vi "Example_MoveWithIPM.vi"() -> ()   [LabVIEW 2018]
doc: "Example how to do a interpolated position movement. Before starts this example the device must be tuned and the parameter settings must be correct.\nThe example shows:\n - how to initialise and close an interface (e.g. USB)\n - define home position to 0\n - sequence of an interpolated positioning (sinus wave untill stop button is pressed)\n - stops the trajectory"
panel:
  in  "stop":bool
  in  "array for PVT values":T1(array[cluster])=[{"position"=1492, "velocity"=203, "time"=240}, {"position"=2891, "velocity"=184, "time"=240}, {"position"=4107, "velocity"=153, "time"=240}, {"position"=5066, "velocity"=112, "time"=240}, {"position"=5706, "velocity"=65, "time"=240}, {"position"=5988, "velocity"=13, "time"=240}, {"position"=5894, "velocity"=-39, "time"=240}, {"position"=5429, "velocity"=-89, "time"=240}, {"position"=4623, "velocity"=-134, "time"=240}, {"position"=3527, "velocity"=-169, "time"=240}, {"position"=2209, "velocity"=-195, "time"=240}, {"position"=752, "velocity"=-208, "time"=240}, {"position"=-752, "velocity"=-208, "time"=240}, {"position"=-2209, "velocity"=-195, "time"=240}, {"position"=-3527, "velocity"=-169, "time"=240}, {"position"=-4623, "velocity"=-134, "time"=240}, {"position"=-5429, "velocity"=-89, "time"=240}, {"position"=-5894, "velocity"=-39, "time"=240}, {"position"=-5988, "velocity"=13, "time"=240}, {"position"=-5706, "velocity"=65, "time"=240}, {"position"=-5066, "velocity"=112, "time"=240}, {"position"=-4107, "velocity"=153, "time"=240}, {"position"=-2891, "velocity"=184, "time"=240}, {"position"=-1492, "velocity"=203, "time"=240}, {"position"=0, "velocity"=209, "time"=240}, {"position"=1492, "velocity"=203, "time"=240}, {"position"=2891, "velocity"=184, "time"=240}, {"position"=4107, "velocity"=153, "time"=240}, {"position"=5066, "velocity"=112, "time"=240}, {"position"=5706, "velocity"=65, "time"=240}, {"position"=5988, "velocity"=13, "time"=240}, {"position"=5894, "velocity"=-39, "time"=240}, {"position"=5429, "velocity"=-89, "time"=240}, {"position"=4623, "velocity"=-134, "time"=240}, {"position"=3527, "velocity"=-169, "time"=240}, {"position"=2209, "velocity"=-195, "time"=240}, {"position"=752, "velocity"=-208, "time"=240}, {"position"=-752, "velocity"=-208, "time"=240}, {"position"=-2209, "velocity"=-195, "time"=240}, {"position"=-3527, "velocity"=-169, "time"=240}, {"position"=-4623, "velocity"=-134, "time"=240}, {"position"=-5429, "velocity"=-89, "time"=240}, {"position"=-5894, "velocity"=-39, "time"=240}, {"position"=-5988, "velocity"=13, "time"=240}, {"position"=-5706, "velocity"=65, "time"=240}, {"position"=-5066, "velocity"=112, "time"=240}, {"position"=-4107, "velocity"=153, "time"=240}, {"position"=-2891, "velocity"=184, "time"=240}, {"position"=-1492, "velocity"=203, "time"=204}, {"position"=0, "velocity"=209, "time"=240}, {"position"=1492, "velocity"=203, "time"=240}, {"position"=2891, "velocity"=184, "time"=240}, {"position"=4107, "velocity"=153, "time"=240}, {"position"=5066, "velocity"=112, "time"=240}, {"position"=5706, "velocity"=65, "time"=240}, {"position"=5988, "velocity"=13, "time"=240}, {"position"=5894, "velocity"=-39, "time"=240}, {"position"=5429, "velocity"=-89, "time"=240}, {"position"=4623, "velocity"=-134, "time"=240}, {"position"=3527, "velocity"=-169, "time"=240}, {"position"=2209, "velocity"=-195, "time"=240}, {"position"=752, "velocity"=-208, "time"=240}, {"position"=-752, "velocity"=-208, "time"=240}, {"position"=-2209, "velocity"=-195, "time"=240}, {"position"=-3527, "velocity"=-169, "time"=240}, {"position"=-4623, "velocity"=-134, "time"=240}, {"position"=-5429, "velocity"=-89, "time"=240}, {"position"=-5894, "velocity"=-39, "time"=240}, {"position"=-5988, "velocity"=13, "time"=240}, {"position"=-5706, "velocity"=65, "time"=240}, {"position"=-5066, "velocity"=112, "time"=240}, {"position"=-4106, "velocity"=153, "time"=240}, {"position"=-2891, "velocity"=184, "time"=240}, {"position"=-1492, "velocity"=203, "time"=240}, {"position"=0, "velocity"=209, "time"=240}]
  in  "IPM buffer parameter":T2={"underflowWarningLimit"=4, "overflowWarningLimit"=60}
  in  "nodeId":u16=1
  in  "communication settings in":T3={"deviceName"="EPOS2", "protocolStackName"="MAXON SERIAL V2", "interfaceName"="USB", "portName"="USB0", "baudrate"=1000000, "timeout"=500}
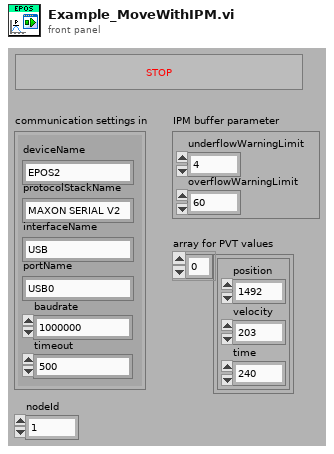
[diagram p1: front panel]
types:
  T1 = cluster{"position":i32, "velocity":i32, "time":u8}[]
  T2 = cluster{"underflowWarningLimit":u16, "overflowWarningLimit":u16}
  T3 = cluster{"deviceName":string, "protocolStackName":string, "interfaceName":string, "portName":string, "baudrate":u32, "timeout":u32}
  T4 = cluster{"position":i32, "velocity":i32, "time":u8}
  T5 = cluster{"trajectoryRunning":i32, "isUnderflowWarning":i32, "isOverflowWarning":i32, "isVelocityWarning":i32, "isAccelerationWarning":i32, "isUnderflowError":i32, "isOverflowError":i32, "isVelocityError":i32, "isAccelerationError":i32}
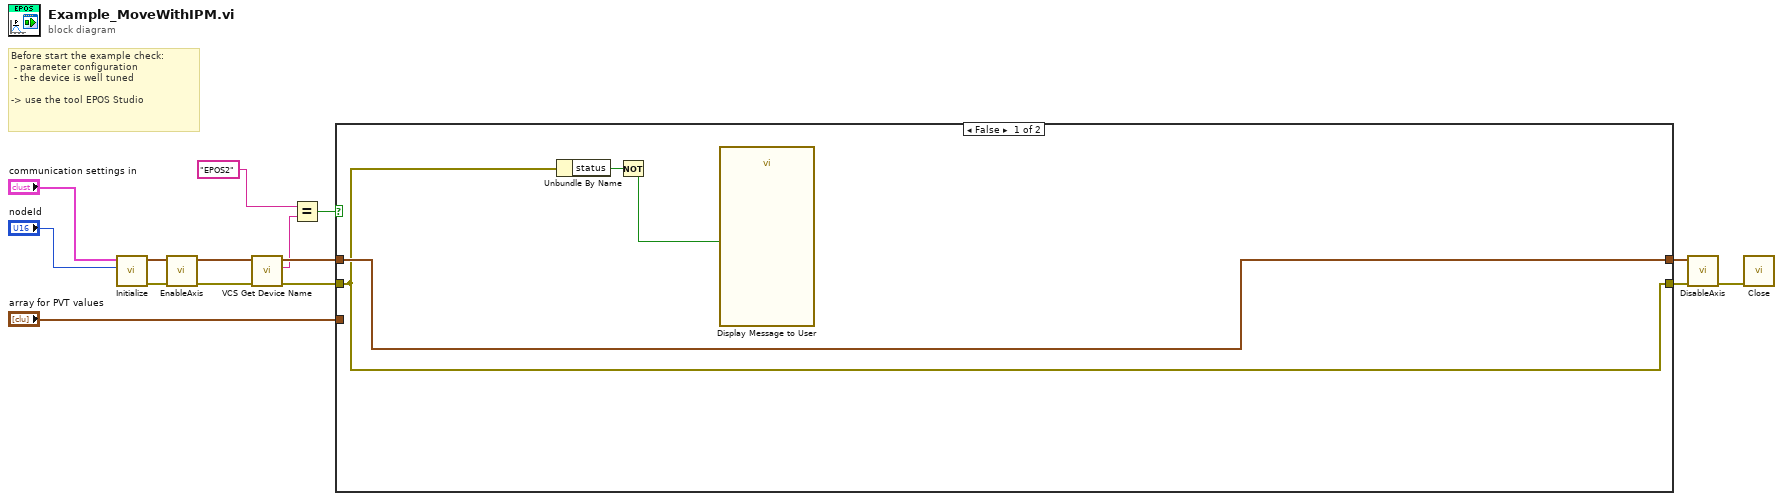
[diagram p0: block diagram]
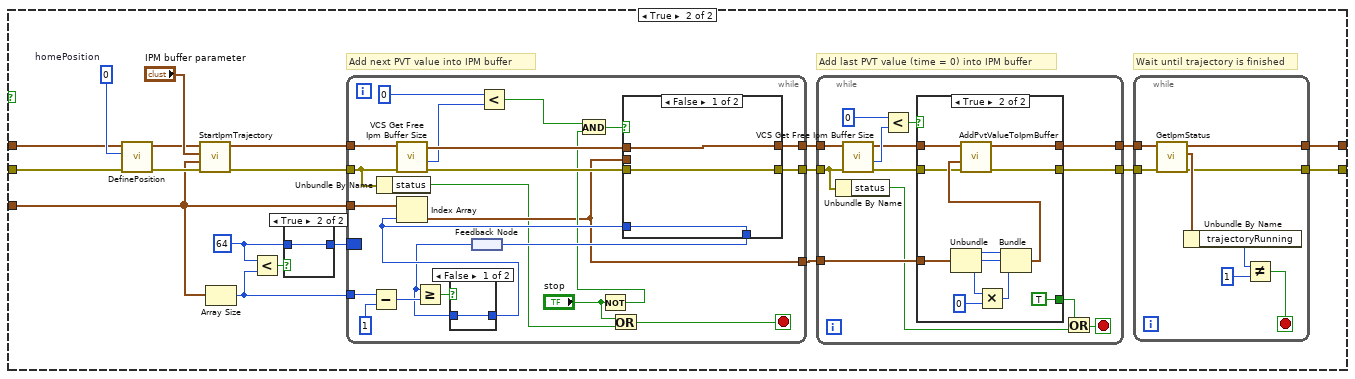
[diagram p2: hidden frame]
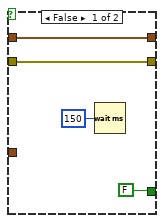
[diagram p3: hidden frame]
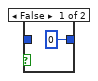
[diagram p4: hidden frame]
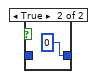
[diagram p5: hidden frame]
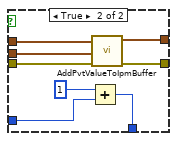
[diagram p6: hidden frame]
diagram:
  # "Before start the example check:\n - parameter configuration\n - the device is well tuned \n\n-> use the tool EPOS Studio"
  n1 = call "Initialize.vi"("nodeId"="nodeId", "communication settings in"="communication settings in") -> ("error out"=w13:errorcluster, "axis out"=w12:cluster{"keyHandle":u32, "nodeId":u16})  [unwired: 8 in]
  n2 = call "EnableAxis.vi"("error in (no error)"=w13, "axis in"=w12) -> ("error out"=w5:errorcluster, "axis out"=w4:cluster{"keyHandle":u32, "nodeId":u16})  [unwired: 4 in]
  n3 = call "VCS Get Device Name.vi"("error in (no error)"=w5, "axis in"=w4) -> ("error out"=w6:errorcluster, "deviceName"=w2:string, "axis out"=w7:cluster{"keyHandle":u32, "nodeId":u16})  [unwired: 7 in]
  n4 = Equal?(x="EPOS2", y=w2) -> (x = y?=w3:bool)
  n5 = case shown="False" w3 {
    tunnel: "array for PVT values" -> [_ w35]
    tunnel: [w17 w28] -> w9
    tunnel: [w16 w27] -> w8
    tunnel: w7 -> [w17 w21]
    tunnel: w6 -> [w16 w20]
    frame False {
      n6 = Unbundle By Name(w16) -> ("status"=w18:bool)
      n7 = Not(x=w18) -> (.not. x?=w19:bool)
      n8 = call "Display Message to User"("Enable"=w19) -> ()  [unwired: 9 in, 2 out]
    }
    frame True {
      w29 = 64 ("x")
      w39 = 0  # homePosition
      # "Wait until trajectory is finished"
      # "Add last PVT value (time = 0) into IPM buffer"
      # "Add next PVT value into IPM buffer"
      n9 = call "DefinePosition.vi"("error in (no error)"=w20, "homePosition"=w39, "axis in"=w21) -> ("error out"=w37:errorcluster, "axis out"=w36:cluster{"keyHandle":u32, "nodeId":u16})  [unwired: 3 in]
      n10 = call "StartIpmTrajectory.vi"("error in (no error)"=w37, "array for PVT values (max. 64 values)"=w35, "IPM buffer parameter"="IPM buffer parameter", "axis in"=w36) -> ("error out"=w33:errorcluster, "axis out"=w34:cluster{"keyHandle":u32, "nodeId":u16})  [unwired: 2 in]
      n11 = Array Size(array=w35) -> (size(s)=w32:i32)
      n12 = Less?(x=w29, y=w32) -> (x < y?=w31:bool)
      n13 = case shown="True" w31 {
        tunnel: [0 ("x") w78] -> w30
        tunnel: w29 -> [_ w78]
        frame False {
        }
        frame True {
        }
      }
      n14 = while {
        tunnel: w35 -> [w101]
        tunnel: w32 -> [w91]
        tunnel: [w99] -> w26
        tunnel: [w98] -> w25
        tunnel: w34 -> [w96]
        tunnel: w33 -> [w82]
        tunnel: [w83] -> w24
        border: w30 -> [_]
        stop <- w79 stop-if-true
        n15 = Subtract(x=w91, y=1) -> (x-y=w95:i32)
        n16 = Unbundle By Name(w82) -> ("status"=w80:bool)
        n17 = call "VCS Get Free Ipm Buffer Size.vi"("error in (no error)"=w82, "axis in"=w96) -> ("error out"=w97:errorcluster, "bufferSize"=w87:u32, "axis out"=w100:cluster{"keyHandle":u32, "nodeId":u16})  [unwired: 6 in]
        n18 = feedback #1() -> (w89:u32)
        n19 = Greater Or Equal?(x=w89, y=w95) -> (x >= y?=w93:bool)
        n20 = case shown="False" w93 {
          tunnel: [w102 u32 0 ("x")] -> w92
          tunnel: w89 -> [w102 _]
          frame False {
          }
          frame True {
          }
        }
        n21 = Index Array(array=w101, index=w92) -> (element=w83:T4)
        n22 = Less?(x=u32 0, y=w87) -> (x < y?=w86:bool)
        n23 = Not(x="stop") -> (.not. x?=w85:bool)
        n24 = And(x=w86, y=w85) -> (x .and. y?=w84:bool)
        n25 = Or(x="stop", y=w80) -> (x .or. y?=w79:bool)
        n26 = case shown="False" w84 {
          tunnel: w83 -> [_ w107]
          tunnel: w100 -> [w105 w108]
          tunnel: [w105 w114] -> w99
          tunnel: [w104 w113] -> w98
          tunnel: w97 -> [w104 w112]
          tunnel: w92 -> [w106 w111]
          tunnel: [w106 w110] -> w90
          frame False {
          }
          frame True {
            n27 = Add(x=u32 1, y=w111) -> (x+y=w110:u32)
            n28 = call "AddPvtValueToIpmBuffer.vi"("error in (no error)"=w112, "PVT value"=w107, "axis in"=w108) -> ("error out"=w113:errorcluster, "axis out"=w114:cluster{"keyHandle":u32, "nodeId":u16})  [unwired: 3 in]
          }
        }
        n29 = feedback-in #1(w90) -> ()
      }
      n30 = while {
        tunnel: w26 -> [w49]
        tunnel: w25 -> [w43]
        tunnel: w24 -> [w46]
        tunnel: [w45] -> w23
        tunnel: [w44] -> w22
        stop <- w42 stop-if-true
        n31 = Unbundle By Name(w43) -> ("status"=w40:bool)
        n32 = call "VCS Get Free Ipm Buffer Size.vi"("error in (no error)"=w43, "axis in"=w49) -> ("error out"=w48:errorcluster, "bufferSize"=w51:u32, "axis out"=w47:cluster{"keyHandle":u32, "nodeId":u16})  [unwired: 6 in]
        n33 = Less?(x=u32 0, y=w51) -> (x < y?=w50:bool)
        n34 = case shown="True" w50 {
          tunnel: w48 -> [w55 w62]
          tunnel: w47 -> [w54 w61]
          tunnel: w46 -> [_ w60]
          tunnel: [FALSE TRUE] -> w41
          tunnel: [w54 w58] -> w45
          tunnel: [w55 w57] -> w44
          frame False {
            n35 = Wait (ms)(milliseconds to wait=u32 150) -> ()  [unwired: 1 out]
          }
          frame True {
            n36 = Unbundle(w60) -> ("position"=w63:i32, "velocity"=w64:i32, "time"=w66:u8)
            n37 = Multiply(x=w66, y=u8 0) -> (x*y=w67:u8)
            n38 = Bundle("position"=w63, "velocity"=w64, w67) -> (w68:cluster{"position":i32, "velocity":i32, u8})  [unwired: 1 in]
            n39 = call "AddPvtValueToIpmBuffer.vi"("error in (no error)"=w62, "PVT value"=w68, "axis in"=w61) -> ("error out"=w57:errorcluster, "axis out"=w58:cluster{"keyHandle":u32, "nodeId":u16})  [unwired: 3 in]
          }
        }
        n40 = Or(x=w41, y=w40) -> (x .or. y?=w42:bool)
      }
      n41 = while {
        tunnel: w23 -> [w75]
        tunnel: [w74] -> w28
        tunnel: w22 -> [w73]
        tunnel: [w72] -> w27
        stop <- w69 stop-if-true
        n42 = call "GetIpmStatus.vi"("error in (no error)"=w73, "axis in"=w75) -> ("error out"=w72:errorcluster, "IPM status"=w76:T5, "axis out"=w74:cluster{"keyHandle":u32, "nodeId":u16})  [unwired: 3 in]
        n43 = Unbundle By Name(w76) -> ("trajectoryRunning"=w71:i32)
        n44 = Not Equal?(x=w71, y=1) -> (x != y?=w69:bool)
      }
    }
  }
  n45 = call "DisableAxis.vi"("error in (no error)"=w8, "axis in"=w9) -> ("error out"=w11:errorcluster)  [unwired: 4 in, 1 out]
  n46 = call "Close.vi"("error in (no error)"=w11) -> ()  [unwired: 10 in, 1 out]
